vi "2023_day19.vi"() -> ()   [LabVIEW 2021]
uses:
  <vilib>/regexp/Match Regular Expression.xnode
panel:
  out "Task 1":i32
  out "Array":cluster{"Array":string[], "Array":i32[]}[](array[cluster])
  out "Rules":T1(array[cluster])
  out "line 2":string
  out "line":string
  in  "Switch":bool caption="Ex. Data  vs.  User Data"
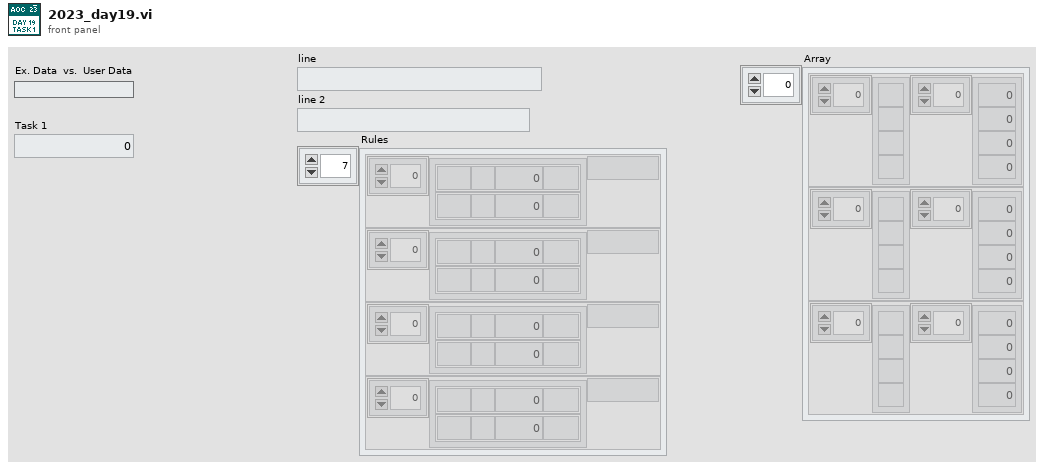
[diagram p1: front panel]
types:
  T1 = cluster{"Array":cluster{"String":string, "String":string, "Numeric":i32, "String":string}[], "String 2":string}[]
  T2 = cluster{cluster{string, string, i32, string}[], "delimiter (Tab)":string}
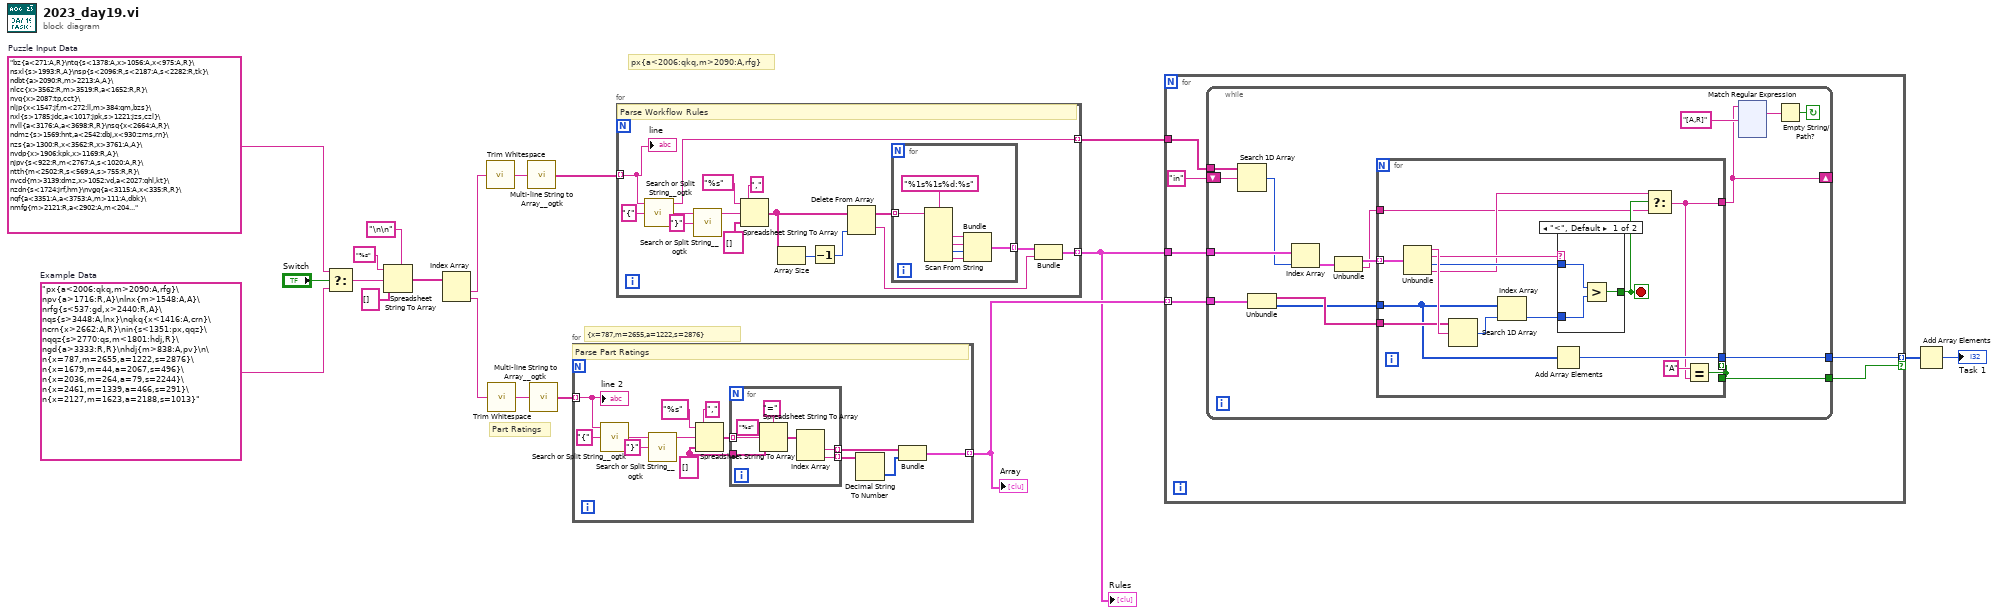
[diagram p0: block diagram]
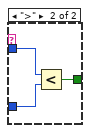
[diagram p2: hidden frame]
diagram:
  w17 = "bz{a<271:A,R}\ntq{s<1378:A,x>1056:A,x<975:A,R}\nsxl{s>1993:R,A}\nsp{s<2096:R,s<2187:A,s<2282:R,tk}\ndbt{a>2090:R,m>2213:A,A}\nlcc{x>3562:R,m>3519:R,a<1652:R,R}\nvq{x>2087:tp,cct}\nljp{x<1547:jf,m<272:ll,m>384:qm,bzs}\nxl{s>1785:jdc,a<1017:jpk,s>1221:jzs,czl}\nvll{a<3176:A,a<3698:R,R}\nsq{x<2664:A,R}\ndmz{s>1569:hnt,a<2542:dbj,x<930:zms,rn}\nzs{a>1300:R,x<3562:R,x>3761:A,A}\nvdp{x>1906:kpk,x>1169:R,A}\njpv{s<922:R,m<2767:A,s<1020:A,R}\ntth{m<2502:R,s<569:A,s>755:R,R}\nvcd{m>3139:dmz,x>1052:vd,a<2027:qhl,kt}\nzdn{s<1724:jrf,hm}\nvgq{a<3115:A,x<335:R,R}\nqf{a<3351:A,a<3753:A,m>111:A,dbk}\nmfg{m>2121:R,a<2902:A,m<2043:A,R}\nbxp{s>3412:A,m<2753:A,R}\nnxn{x<672:A,m>2353:A,R}\nhpr{a>1842:A,a>728:hcz,x>1243:A,A}\ncvl{a>669:mjv,m>2629:sc,rdf}\nkxx{a>766:R,a<292:R,A}\ndmg{s>2102:A,s>2014:A,A}\nrgv{a<3593:A,A}\nchn{a>2598:cbs,s>174:A,a<2260:tx,R}\nxz{m<1473:A,x>3212:R,x<2650:A,R}\ngzf{x>339:R,s>2706:R,A}\nzsr{a>3599:R,m>3283:R,s<1003:R,A}\nkc{m>1743:A,a>1102:R,x<2016:A,A}\nfns{s>2718:R,m<250:R,zz}\nrks{x>1085:A,a<3193:R,R}\ntsb{x>2609:R,R}\njpk{a<367:lmr,lkr}\nzt{x<728:A,x<1273:A,x<1612:A,R}\nsm{s<2016:R,m>3494:R,R}\nlqv{x>2509:rgv,mdj}\nqgc{s<2535:A,A}\nmn{x>711:R,R}\nqj{m<2321:A,a>1060:A,m<2640:A,A}\nlvl{x>2318:R,x>1150:R,R}\nfvj{x>629:xm,m>434:tg,R}\ndrm{x>3363:A,s<67:A,m<966:A,A}\nhc{a>2875:R,a<2355:R,A}\nrzh{x<2577:rt,a<1217:zjs,a<1672:A,xt}\nbcf{m<75:tm,s>2347:A,cjj}\nxsd{m<124:A,s>2385:A,bsn}\ndx{m<1166:R,A}\ncsf{s<815:sxq,a<2075:dck,ndb}\ndt{s<3903:R,a>3046:R,A}\nxbj{a<2484:bp,x>3289:rfz,s>239:vs,xs}\njmg{a<3045:pxt,lp}\nmpz{x<1593:R,x>3044:R,a<3808:A,A}\nlhp{x>1339:R,s<2653:A,x>649:R,A}\nll{s<3281:R,A}\ndcq{x>3360:R,m<3027:R,R}\nppg{m<541:R,m>559:R,x<2390:R,R}\nmbz{m<3495:R,s>2446:rks,A}\ncd{m<1335:A,m>1438:A,R}\nkrc{x<733:mfg,a>2761:qh,x>953:dch,zp}\nlvg{m>972:kz,x>495:hzn,a>3117:A,A}\nzhs{m>2206:rf,a<835:A,a>1165:R,R}\nfsh{x>2167:A,s>849:R,R}\nkbr{m<611:cpv,dp}\nrmx{a<1561:rs,s<1865:vq,m<710:tbz,fvq}\nhnh{s<2247:A,s>2348:R,m<339:R,R}\nhzq{m>626:A,a<2948:A,s<2726:A,R}\nrx{s<2136:A,s<2240:R,m>2747:A,R}\nqm{m>429:A,a>2633:dzg,a>2161:A,R}\nsbn{m<3741:R,m<3839:A,s<1462:A,R}\nlpk{s<3389:R,A}\npxt{a>2883:hzq,zh}\nfvq{s>2926:dvb,vmx}\nrz{s>425:md,s<168:pn,R}\nhxn{x>439:R,a<1407:A,A}\nqpg{m>3129:R,R}\npb{a>1824:vzm,x>3183:spc,qmb}\ndvj{a>925:R,s<234:A,R}\nksm{m>1071:A,m<396:A,s<327:A,R}\nqd{m>2276:R,s<225:R,x>3486:R,R}\njzs{m<2895:prh,s<1539:R,a>1512:ktn,zs}\ndp{x<1710:A,m<665:R,a>3405:R,R}\nfnf{s>2544:A,m<2240:R,A}\nfk{a>767:A,m<2071:R,R}\nndq{x<581:vr,a>2446:qjm,s>2111:jl,dhs}\nkkl{s>2054:R,m<3499:R,m<3761:R,cjk}\nxtv{a>1875:A,x>3752:R,m<2351:A,A}\nxpf{s<1203:nr,m<3594:vn,x<2455:A,sbn}\nhfx{a<1359:R,s<449:A,s>777:R,A}\nmrm{a>1753:tpl,x>1066:zzk,glm}\nnxx{s>2462:gxf,jz}\nqsf{a>2892:R,A}\nxt{s<1927:R,s<2188:A,a>1886:A,A}\nvbm{a<1287:A,xsj}\ncdh{a>2648:dq,vtq}\njc{m>2325:R,x<465:A,m>2139:A,R}\nzzk{a>1062:xg,m>3439:vf,lg}\nfvl{s>3488:R,a<3070:A,A}\nkdk{m>2643:gl,qd}\nbhd{x>1591:R,a<3099:R,R}\njdc{s<2074:dsl,m<2676:gc,A}\ngz{x>960:A,vgq}\nps{m>337:A,A}\nclf{s<1430:ct,nk}\nbsn{a<2452:R,s<2072:A,a<2687:A,A}\nfjr{s>918:zsr,m<2877:A,R}\nbx{m>3430:R,A}\nzg{m>1485:A,s>2852:A,m<1298:R,jrq}\nlp{x<1690:A,s>2595:R,x>2670:A,R}\nqmb{x<2671:lnl,s>696:R,A}\njk{s<1930:R,x<2990:R,R}\nlx{a<2583:dz,mbc}\npkq{s<368:R,s>527:R,a>3711:A,R}\nrzl{m>1462:A,s<2457:A,s<2597:R,R}\ntgr{a>2640:R,R}\npj{x>2209:xp,a>2278:A,mt}\nlmr{s>1359:R,x<3503:R,A}\nnq{x>1084:R,x>478:R,A}\nndb{a>3110:ss,x>3077:gmd,s<1734:fn,js}\nvpg{x<706:fdp,a>852:hfx,a<542:A,A}\ngxn{a<312:lsk,x>2287:dj,A}\ntcl{a>1665:A,zzr}\nsjk{x>3226:A,A}\nfkb{m>2795:jk,a<3439:jq,x>3038:R,bzr}\npl{m<1045:A,s<3912:A,x<2819:A,R}\nhhj{a>2420:R,s<2764:R,a<2288:R,A}\nsqb{s>1984:rx,R}\nqbd{m>2065:A,x<882:A,m<1999:R,A}\ngxv{m>595:R,a>3447:ppg,x<2625:R,fpx}\nbf{a<3541:R,drm}\nzjs{s<1967:R,s>2205:R,R}\ncct{s<720:hj,jqg}\nsqr{s<815:R,m>3766:R,s>962:A,A}\ndsl{a<888:A,m>3114:A,R}\nhg{a<3188:A,a<3272:A,R}\ngn{m<348:A,a>3297:R,A}\ncrq{m<369:cdk,x>1901:lh,gz}\nzzr{a>1577:R,s<2759:A,s>2978:A,R}\nsdq{s<2531:ft,nbf}\ncx{s<2002:A,A}\nzch{m<3110:A,a<580:R,A}\njm{a>3202:A,tth}\ntpl{m<3521:rp,s<417:chn,vgg}\nlsk{s<2835:A,a<146:A,A}\nkt{s>1824:gj,m<2677:jxf,gcz}\nvdb{s<2725:R,A}\nkrk{m>1118:A,x>3794:A,s<2745:A,A}\nhx{s>3398:R,s<3375:R,x<1299:A,A}\nmbc{x<3258:R,a>3221:R,x>3540:A,dcq}\nbcq{s<707:vvf,m<463:rv,A}\nvf{x<1370:R,s<575:A,sqr}\nmk{m>2037:tfj,x>1441:A,s<2719:A,A}\nktn{a>1844:R,x<3658:A,s>1639:A,R}\nhkh{s<3644:qnf,a>2509:R,a<2158:jg,sj}\nqkb{s>221:A,A}\nnbf{x>1635:A,R}\nktf{s<1930:jff,a>729:sv,s<2195:R,R}\ntbz{s>3054:hjn,m<295:ts,m>474:sf,rtk}\nrg{a>2237:A,s>2763:R,R}\ntn{s<2624:mq,vdp}\nzx{s<2597:R,R}\nhp{s>3853:dt,s<3725:nss,tgr}\nkkh{a>2790:R,m>189:A,R}\npmb{m<257:R,R}\ntx{s>78:R,a>2050:R,R}\nzhq{a>1619:A,x<2261:R,R}\nqh{m>2162:R,m>2032:A,R}\nsfh{s>3658:R,A}\nxs{x<2780:R,A}\nmv{a<2521:hd,gxv}\nzl{x>2215:cd,m>1293:hq,xv}\nqc{s<1635:A,A}\nvb{x>631:vkd,s>2815:xn,s>2755:A,gzf}\nlv{s>3494:A,A}\nlj{a<2530:A,m>36:R,A}\nkz{x>572:R,a<2969:R,A}\npnb{m<81:ljx,xsd}\nrv{s>1327:A,A}\nnkl{x>2711:R,x>2565:R,A}\ndkn{a<1500:pfp,x>1968:dtr,cpb}\nsz{m<2803:cfx,mbz}\nvm{s>3556:xtv,fg}\nvqr{a<2337:A,s>2233:R,R}\nss{s>1468:fkb,s<1048:fjr,x<3082:qfl,cjz}\nfp{a>2830:A,s<2169:R,R}\nrjr{m>1228:R,R}\nkl{a>644:A,R}\nzlb{x<1411:qf,a>3522:bcf,nxx}\nckr{m<2196:qbd,x>784:R,mxv}\nhb{m>2153:R,R}\nnml{x<1589:qv,sxk}\nqr{m<2677:A,s>2608:R,m<3452:A,A}\njh{s>1262:glg,m>2684:A,R}\nkh{m>2680:A,m>2361:R,A}\nvr{x<257:R,xhv}\nhjn{m>467:mv,s>3603:hp,ljp}\nfq{m>2822:tv,x<2595:nml,x<3261:tt,rfp}\nvtq{x>2240:xz,s>3083:A,dh}\ngb{s<2899:bz,tb}\nmrd{x>1271:lr,m<2641:rm,x<526:zqr,fs}\nmld{a>2486:A,x>3111:R,m<316:A,R}\nhcc{a<1236:A,a<1350:A,zlx}\nfs{s>603:R,A}\ncjz{a>3524:R,fjh}\npjk{a<2164:R,s<3627:R,x<2770:A,A}\nmxv{x<464:A,R}\nmjv{a>987:xhn,vtt}\npfc{s<3515:R,m<2266:A,s<3692:R,A}\ntz{m>914:kkg,a<2667:rng,x<1472:rq,gn}\nqhl{s<1607:jkc,a>1133:mds,nt}\nqg{s>1998:R,x<2415:A,R}\ndl{s<2694:ghj,x>2629:xpd,lqs}\nvgg{a>2972:R,zt}\nvqd{s>1429:A,x>354:A,A}\nqfh{s>3793:xpb,x<2138:hkh,a>2637:vg,hv}\nvmx{s>2326:dl,x>1382:dpd,m>1421:ndq,vrf}\nxsj{m>2720:R,a<1313:R,a>1330:A,R}\nnps{a<2079:R,m>1380:R,a>2173:kf,A}\nkxp{m<1582:A,A}\njln{m<1242:A,a<2086:R,a>2252:A,A}\ntfj{a>392:R,x>1464:A,x<774:R,R}\nghj{m<1275:vnz,m<1584:rzl,m<1710:hc,lvl}\njmb{s>2167:R,s>2124:R,R}\njg{x<1043:R,R}\ngc{m>2288:R,x>3485:R,A}\nlch{m>981:A,x<307:A,A}\ndch{m<2204:R,a>2068:R,R}\nfj{a<855:zg,gvv}\nhv{m>1308:pjk,a>1953:R,m>961:R,sfh}\ntv{a<1389:ctq,pj}\nqt{m>3033:ktf,m>2364:sqb,rzh}\ndhs{m<1658:A,s>1977:sft,x>884:R,xdl}\nbld{x<2869:A,R}\nlh{m<436:dbl,a<2712:lq,m>457:A,A}\nhvh{s<242:R,m>1756:hqt,x<1329:A,dzs}\nzb{x<902:R,s>341:A,s<172:A,R}\nmd{a>3376:R,R}\nzlx{s<733:A,R}\nxcl{a>870:A,m>3355:A,a<455:R,R}\nvmn{s<2480:A,R}\nhqt{a<526:A,m>1813:A,R}\ntnp{s<1812:R,bgn}\nljx{x<2542:lhp,lj}\npg{x<1652:R,R}\nvd{x<1464:hpr,x<1655:tnp,sxn}\nzh{m>578:A,a<2830:A,R}\ndzs{x>1651:A,A}\nsj{s<3698:R,m<1133:A,A}\nks{a>1809:A,R}\nxpb{x<1450:R,m>1232:zq,pl}\nffg{x>2163:lt,s>3351:hx,x>786:qnr,lch}\ndnn{m<2585:R,A}\ngmd{x<3605:zdn,gct}\njq{x<2628:A,A}\ncpv{s<2035:R,R}\ngct{x<3764:A,x>3852:R,a>2497:hl,A}\nvlc{x>2214:A,s<3472:R,s>3806:A,A}\nbvl{m<2738:R,R}\nvxf{m<3019:A,x<3541:A,A}\ntg{a<3439:R,s<2677:R,R}\nfsf{a>2519:A,R}\npv{a<420:A,m>1733:A,R}\nfff{a>2742:A,x>3397:A,A}\nlb{s<2419:A,s<2498:R,a<1250:A,R}\ngfp{x>3062:A,A}\ncjj{a>3731:R,A}\ndqf{s<2041:R,a<2123:A,vpk}\npc{x<2498:R,s>2942:A,R}\npsb{m<380:A,m<422:rjp,R}\nxhn{m<2996:qj,a>1071:cn,a<1022:R,hgp}\npt{a<2754:nkl,A}\nzjz{a<734:A,R}\npm{x<1100:A,m>2655:R,a>3140:R,A}\nrdf{m>2278:gxn,x>2317:cvv,mk}\ndts{x>1531:pg,a<3446:vj,m>1041:kq,pkq}\ndck{x>3214:xl,s>1666:qt,nsj}\nlc{x>361:A,A}\nkkg{m>1303:A,a<2452:A,x<1273:R,R}\nvg{x>3184:A,m<1418:R,x>2660:bld,A}\njt{x>2477:R,a>2635:zx,fsf}\nhm{a>2487:A,a<2274:A,m<2628:R,R}\ngdf{a>1833:A,m>2601:R,x>3693:A,A}\nbn{s>2146:A,R}\nmds{a<1669:kh,ks}\nkjs{m<1076:bg,x<2959:sq,a>2348:jzk,nps}\ntpd{m>3019:R,m<2929:zjz,dhm}\nvj{a<3135:R,A}\nin{m<1904:rmx,dv}\nbg{x<2803:zk,A}\nkq{s>335:R,x<1444:R,s<144:R,R}\ndh{m<1504:A,x<1117:R,R}\nglg{s>1491:A,a>2699:R,x<2115:R,R}\ngq{m>582:A,s>2494:R,R}\nczl{m>3218:lcc,a>1482:gdf,s>1070:R,jpv}\nfb{x<798:A,m<1278:A,x<1320:A,R}\nbgn{m<2676:A,x>1552:A,a<2102:A,R}\njkc{s>1316:lvr,A}\njff{s<1814:A,A}\npfp{a>1356:lk,s<2593:lb,vbm}\nhzn{s>291:A,m<350:R,s>107:A,R}\nnss{x>1361:R,m<275:R,A}\nmt{a>1794:A,a<1619:A,R}\ncbs{x>749:R,x>452:A,R}\nzp{a>2382:R,m>2160:A,A}\ncdj{m<1426:A,m<1470:R,R}\ngkc{a>3431:A,m<2719:R,R}\nrng{a<2253:A,s<1364:A,A}\ncm{x<701:A,s<2077:R,R}\nsl{s>218:A,a<1428:R,R}\nlr{s<676:dnn,m<2639:R,tkc}\nqrj{a>3647:A,R}\nqfl{x<2572:pf,x<2780:R,a<3582:A,lzt}\nkd{a>2021:R,x<3445:R,A}\nhth{a<436:bj,a<537:A,a>618:rd,zch}\nvtp{m>2029:fk,s<186:A,fv}\nlk{x>1877:R,x<1197:hxn,s>2758:mg,qr}\nfjh{s<1233:A,s>1369:A,A}\nbl{x>3051:kdk,m>2606:cs,x>2593:qkb,dqk}\njxc{s<754:A,s<919:R,x>326:R,A}\nsh{m<1271:ffg,x<2154:lpk,ml}\nrvk{a>1716:jb,m>2310:mrd,x<929:bsr,mtv}\njz{s<2076:A,R}\ngxf{m>119:R,R}\ntm{s>2460:R,s<2108:A,R}\nhs{a<1050:A,s>1331:A,A}\nklm{m>334:A,a<3340:hg,mn}\nvrf{x>831:qn,jss}\ntk{x<714:R,m>536:A,A}\ngcz{x>689:fgq,a>2814:R,a>2515:R,R}\nvrc{a>617:hcc,bcq}\nfv{x<323:A,a>731:R,m<1985:R,R}\nqv{s<3495:nxn,ntn}\nzqr{s>620:R,a>1126:bvl,a>521:klf,pht}\nhcz{m>2716:R,a<1342:A,s<1707:A,R}\nxn{s<2868:R,A}\nph{a<420:A,x<2533:R,a<671:R,A}\nbp{a>1918:A,x<3035:rjr,m<1071:xzr,R}\nzdf{a>958:A,pv}\nhgp{a>1049:R,R}\nmq{m>638:A,s<2293:A,a>616:pmb,ql}\ncn{s<2663:A,R}\ndhm{s>353:A,R}\njzk{s<568:R,x>3650:A,s>707:R,R}\ncjk{x>2540:R,s>1858:A,m>3890:A,A}\ncrx{m>562:gq,x<1668:mf,x<2473:R,qgc}\nbjh{s>952:A,R}\nfxm{x<480:R,a<2492:A,x>663:dtc,cdt}\nvfp{x<2978:R,s<2782:R,bx}\nklf{s<297:R,A}\nrm{a<641:vv,R}\nflb{s<2029:R,A}\nvnz{a>2624:A,R}\nfth{m<3233:A,x>2427:A,a<1264:R,R}\nqzc{s<2056:fd,x<2546:jmb,fp}\nxzr{a<1702:A,x<3487:R,R}\nspc{x<3466:A,R}\nrvs{m<2531:R,s<732:R,a>1885:R,A}\nbj{x<2674:R,x<3312:A,R}\nctq{x>2179:ktg,xcl}\nljf{a>2607:R,A}\nsxk{a<2523:vlc,a<3269:nlv,pfc}\nvkd{m<3011:R,A}\nfpx{x<3400:R,m<513:A,m<550:R,A}\njvz{x<2305:R,R}\ntp{s>785:clf,a>3143:fc,s>403:kjs,xbj}\nbzr{x>2399:A,A}\nct{s<1142:R,m>1072:cxn,m<576:R,R}\ndpz{x<2890:R,m<1145:R,m>1208:A,R}\ntdk{s<953:R,s<1004:A,A}\nvvf{a>308:R,R}\nmdc{s<545:A,R}\nzms{s<1338:vt,vqd}\nsxq{s<539:bl,pb}\nnpq{a>1733:A,s<2028:R,A}\nst{s>1119:kkn,a<1471:fth,a>1798:A,A}\nqgx{s<2114:qg,x<2550:dx,kd}\ntkc{s<834:A,s>935:R,s<888:A,R}\nvn{a>368:A,x>2719:R,a<186:A,R}\nhdj{m>1379:R,a<3199:A,R}\nfdk{s>760:R,s<721:R,R}\njss{x<523:A,m>949:ljf,cf}\nhfj{m<2440:R,A}\nxmq{s>721:A,A}\nglr{s<409:R,a>2481:vx,a<2006:rvs,R}\npn{s>103:A,x<1962:R,x<2041:R,R}\nrbn{m>1175:A,x<1104:R,A}\nkxh{s>260:A,R}\ngj{x<583:R,R}\nxhd{m>1531:A,x<2769:A,A}\nln{x>1465:R,m>3662:R,A}\nkj{a>2600:R,a>2074:R,a<1875:A,R}\nrds{s>3324:R,m>318:R,A}\ndg{s<1209:R,x<1771:A,a<1172:R,R}\ndj{m>2401:A,x<3015:A,R}\nxcs{m>1181:A,qrj}\nnr{x>2543:R,R}\njrf{s<1411:A,x>3427:A,a>2442:A,A}\nmm{x<803:R,x>1048:A,R}\nts{m>185:nz,a<3026:pnb,zlb}\nnz{a>2521:jzb,s>2272:fns,dqf}\njqg{x>791:tz,fxm}\nrfz{m<1244:R,m>1510:A,m<1357:A,cdj}\nmg{a<1429:A,A}\nlld{a<2189:R,x<1847:R,x>3023:A,A}\nfql{a>1962:A,A}\nfc{s>306:xcs,s<188:bf,a>3705:kxh,knl}\nqhm{a>3166:R,x<2392:R,s>2102:A,A}\nbzs{s>3380:vll,s<3197:tsb,s>3273:rds,mld}\nxxf{x>1829:lx,s>2658:ljc,sz}\nmf{a<3800:R,A}\nnk{a>2593:qc,hxg}\nxsx{a<1715:A,a<1733:A,R}\nsf{s<2353:fx,a<2799:cgr,a>3459:jj,jmg}\nlg{a<481:R,m<3125:mdc,A}\nlqs{s>2841:A,x>1238:A,a>2711:R,rg}\ncdt{s>1120:R,s<974:R,m<793:R,A}\ncgr{a>2377:jt,fql}\nvv{m>2422:R,A}\npht{x>323:R,m<2739:R,s<391:A,A}\nfd{s<1901:A,x>2345:R,R}\nqnf{x>1052:A,A}\nslf{x<2902:A,x<3031:hb,a>1612:xb,R}\nrp{a<2688:qpg,s<561:zb,s>820:bjh,xmq}\nxp{x<3009:A,s>3497:R,R}\nsc{s<2609:vmn,x>1372:hth,gb}\nxb{x<3182:R,m>2184:A,m<2037:R,R}\nntn{m>2269:A,A}\nvpk{a<2369:R,m<252:A,x<2607:A,R}\nvx{m<2559:R,R}\nrjp{s<2679:A,a<2465:R,s<2825:A,A}\nms{m<1237:dg,a>1188:R,s>1186:hs,fsh}\nvt{a>3078:A,m>3607:A,s<1211:R,R}\ndf{m<2520:A,A}\nsft{a>1928:R,A}\nhq{x>1359:R,m>1393:R,R}\ndd{s<3456:jlj,A}\nfph{s>1556:fj,s<564:ls,m<1556:hxz,zmf}\nrs{m<1078:srt,fph}\nktg{s>3470:R,R}\nzk{m<406:R,a>2584:A,R}\nqjm{m>1597:A,s>2130:vfr,m>1500:cx,sxl}\nzz{s>2430:A,A}\njl{m<1587:A,a<2096:R,a<2280:R,vqr}\nvmt{m<3197:R,x<2588:R,x<2868:sm,R}\nbk{x<2404:A,x>3166:R,A}\nmdj{x<1270:A,A}\ngk{x<2248:A,x<2842:A,A}\nnt{m<2598:jc,x<407:A,s>1913:cm,R}\nzkj{m<2762:qsf,s<609:R,mm}\nfgq{x<850:A,a<3052:A,A}\nvfr{a>3009:R,A}\nxm{a>3477:A,m>406:R,x<960:A,R}\nkkn{x<2769:A,a<1377:R,x<3030:A,R}\ncf{x<659:R,x>729:A,A}\nzmf{x>1721:zdf,rfj}\nxpd{x<3509:R,s>2838:A,krk}\ncq{m<808:A,s>2073:A,R}\nxg{s>399:A,x>1421:A,sl}\nlt{m<933:A,s<3372:R,s>3403:R,R}\nrf{m<2272:A,a>1003:R,s>202:A,A}\nbqd{a<3165:kj,rql}\nlms{a>1748:A,s>2636:xsx,m<2315:R,df}\nlkr{x<3666:R,R}\ndvb{s>3461:qfh,s<3266:cdh,sh}\nlvr{x<596:R,a>821:R,R}\nxhv{s>2049:A,A}\nxdl{s>1934:A,a<2067:R,s>1892:A,A}\ndbl{s>2134:R,s<1998:R,R}\nsrt{s>1912:tn,vrc}\nzq{x<2350:R,m<1616:R,A}\nzpc{m<3078:nq,R}\nql{x<2222:R,a>217:A,m>243:R,A}\ncs{m<3468:A,s<268:R,s>406:shg,nrp}\nkp{a<604:R,A}\njzb{a<3429:A,A}\nls{x>2029:xhd,m>1549:hvh,tf}\nqnr{m>1000:A,R}\ndq{s<3056:hdj,s>3189:gk,m<1420:A,A}\ntb{s>2981:R,m<3206:A,A}\nglm{m>3351:vpg,tpd}\nqsm{m<1972:A,m<2023:A,s<2691:A,R}\nft{x<2027:A,x>2763:A,R}\nrn{x>1317:bhd,x<1173:tq,A}\ndqk{x>2356:dbt,x>2136:zhq,a>1610:R,A}\nnv{x>1361:bqd,a<2999:psb,m>357:fvj,klm}\njxf{m>2189:hfj,A}\njs{a<2660:vmt,m>3052:kkl,qzc}\nkpk{x<3286:A,x>3662:R,R}\nqn{s>2152:R,s>2016:rbn,A}\nkf{s>585:A,m>1213:R,A}\nknl{x>2896:R,jr}\nprh{a<1460:A,A}\njrq{a<426:R,a>638:R,R}\ngl{x<3393:A,s<287:A,A}\nfdp{x>267:A,s>393:R,A}\nbsr{s>376:ncs,m<2142:vtp,zhs}\nshg{s<469:A,x<2595:A,R}\nctz{m<2081:fdk,kxx}\nnl{s<2520:A,m>2555:A,x<3105:R,R}\nsxn{a>2415:gkc,R}\ndbj{a>1076:R,a<489:R,A}\nljc{s<2911:vb,zpc}\nfmg{x<1058:bn,a<2339:R,x>1297:A,A}\nrfp{x<3517:dd,vm}\npx{a<465:A,a>714:A,R}\ndzg{s>3282:A,s<3184:R,s>3219:R,A}\nlq{x>3134:A,R}\nxv{s<919:A,a>320:R,s<1148:A,R}\ndtq{x<2179:A,x>2391:ph,A}\nlzt{s>1227:A,R}\nrq{m<349:A,A}\nrtk{s<2469:crq,nv}\ndv{s>2329:pqs,x>1932:csf,zn}\nvs{x<2598:ksm,qcr}\ndpd{a<2738:qgx,m>1283:bbc,ffl}\nrt{s>1987:R,m>2159:R,m>2063:A,R}\ndtc{x<745:A,a>3398:A,m<1224:A,R}\nrfj{s<990:kl,A}\nrd{x<2353:R,a<648:R,x>3265:A,R}\nxdm{x<1258:R,x>1548:A,R}\nrmg{a>1998:R,s>2112:A,flb}\nbv{s>774:R,x<3030:A,R}\nfn{x>2408:pt,jh}\ntt{m>2448:kbj,slf}\ndz{a<2220:A,hhj}\nml{x>2990:fff,a<2565:R,kxp}\nhd{m<570:lld,a<1904:lv,x<1590:A,bk}\nhxg{x<3092:A,m>1196:R,s<1660:R,R}\ncxn{x>3190:A,m<1403:A,s>1314:A,R}\njb{x>1245:jm,m<2402:krc,m>2698:zkj,glr}\npf{s<1266:A,m<2902:R,x>2251:R,R}\nhj{x<1378:lvg,a<2521:jln,x>1817:rz,dts}\ncpb{m>3169:dnk,m<2567:ckr,tcl}\ndbk{m<56:R,x>700:A,a>3875:A,R}\npqs{s>3117:fq,a>1848:xxf,a>1154:dkn,cvl}\nnlv{a<2823:A,a>3076:R,a>2987:R,R}\nvtt{a>783:vdb,m<3188:R,s>2709:pc,A}\nfx{a>2764:kbr,x>1635:rmg,m<589:sp,fmg}\nnrp{a<1932:A,x>2604:A,a>3260:A,A}\nsv{x>2615:R,s<2155:R,A}\ncvv{m<2065:qsm,s<2757:R,R}\ngvv{m<1550:R,kc}\nhl{m>3176:A,x<3803:A,R}\nrql{x>2295:A,s>2830:A,A}\njf{s<3352:kkh,m>311:R,m<107:fvl,R}\nhxz{a>804:ms,zl}\nncs{x>559:A,m>2043:lc,a<640:A,jxc}\njlj{s>3247:A,A}\nffl{m<928:cq,a>3573:dpz,m>1062:A,qhm}\ncfx{m<2449:fnf,pm}\nbbc{m>1669:A,m<1442:jvz,x<2353:dmg,gfp}\nfg{x<3812:R,m>2492:A,A}\njr{a>3444:R,a<3293:R,A}\ndnk{m>3704:xdm,A}\ndtr{m>2899:vfp,a>1679:lms,knr}\nnsj{a>1009:st,m>2813:xpf,x<2635:dtq,px}\nlnl{x>2417:A,A}\nhnt{x<1231:npq,ln}\ntf{a>536:dvj,fb}\nqcr{x>3055:R,A}\nkbj{m<2677:A,bxp}\njj{s>2662:mpz,m>609:sdq,a>3669:crx,lqv}\nmtv{s<699:kp,s<859:ctz,tdk}\nvzm{s>714:bv,s<612:A,x<3205:R,vxf}\nzn{s>1050:vcd,m<2850:rvk,mrm}\ncdk{x<2570:hnh,a>2692:R,s<2088:A,ps}\nknr{s>2839:sjk,s>2584:A,s<2459:A,nl}\n\n{x=1464,m=163,a=691,s=469}\n{x=61,m=72,a=436,s=2532}\n{x=358,m=100,a=2631,s=347}\n{x=266,m=439,a=1250,s=358}\n{x=81,m=2110,a=30,s=86}\n{x=1224,m=758,a=1133,s=881}\n{x=1391,m=3763,a=16,s=2076}\n{x=1149,m=1148,a=126,s=3270}\n{x=214,m=590,a=492,s=818}\n{x=1305,m=687,a=737,s=90}\n{x=20,m=75,a=868,s=847}\n{x=1588,m=99,a=2314,s=998}\n{x=360,m=1002,a=33,s=164}\n{x=68,m=1589,a=992,s=691}\n{x=740,m=2150,a=691,s=668}\n{x=2165,m=707,a=1189,s=161}\n{x=158,m=53,a=416,s=1124}\n{x=601,m=217,a=962,s=623}\n{x=2,m=1314,a=1150,s=357}\n{x=2931,m=1911,a=54,s=1046}\n{x=1037,m=1,a=78,s=974}\n{x=2460,m=689,a=1003,s=1253}\n{x=1793,m=1250,a=331,s=306}\n{x=243,m=247,a=156,s=146}\n{x=1380,m=1600,a=387,s=1362}\n{x=35,m=1900,a=38,s=411}\n{x=349,m=118,a=2452,s=143}\n{x=1314,m=2751,a=1835,s=1569}\n{x=51,m=950,a=1436,s=376}\n{x=347,m=2004,a=11,s=537}\n{x=490,m=576,a=484,s=3066}\n{x=1,m=891,a=3506,s=446}\n{x=1994,m=519,a=644,s=1335}\n{x=2230,m=1165,a=391,s=630}\n{x=1606,m=853,a=1668,s=371}\n{x=904,m=602,a=632,s=1969}\n{x=583,m=794,a=2018,s=851}\n{x=938,m=373,a=1253,s=104}\n{x=704,m=514,a=617,s=525}\n{x=366,m=1662,a=33,s=314}\n{x=753,m=1002,a=285,s=170}\n{x=959,m=2924,a=65,s=1249}\n{x=222,m=701,a=8,s=610}\n{x=887,m=350,a=209,s=3369}\n{x=467,m=137,a=80,s=267}\n{x=671,m=1325,a=928,s=2499}\n{x=69,m=1915,a=539,s=277}\n{x=119,m=2442,a=482,s=495}\n{x=339,m=2398,a=1553,s=1128}\n{x=1364,m=1330,a=1025,s=1678}\n{x=527,m=325,a=341,s=602}\n{x=309,m=1764,a=2066,s=1672}\n{x=772,m=102,a=110,s=723}\n{x=407,m=1522,a=2722,s=26}\n{x=286,m=426,a=863,s=1849}\n{x=483,m=1557,a=1569,s=74}\n{x=487,m=3225,a=2582,s=2012}\n{x=46,m=39,a=650,s=2371}\n{x=98,m=1618,a=1354,s=1140}\n{x=143,m=1488,a=2612,s=3212}\n{x=1894,m=6,a=301,s=2723}\n{x=880,m=50,a=1989,s=1331}\n{x=899,m=308,a=3250,s=1097}\n{x=6,m=235,a=868,s=246}\n{x=128,m=1556,a=1238,s=746}\n{x=561,m=1864,a=743,s=17}\n{x=1170,m=525,a=473,s=2178}\n{x=1927,m=581,a=164,s=1762}\n{x=2467,m=1688,a=258,s=223}\n{x=91,m=80,a=2047,s=1}\n{x=592,m=261,a=374,s=2523}\n{x=1624,m=507,a=3574,s=2063}\n{x=1299,m=696,a=861,s=2958}\n{x=521,m=188,a=1693,s=1079}\n{x=184,m=570,a=1080,s=3064}\n{x=895,m=188,a=714,s=93}\n{x=488,m=123,a=4,s=1884}\n{x=174,m=231,a=499,s=2306}\n{x=1309,m=1190,a=629,s=1364}\n{x=3901,m=1901,a=3133,s=806}\n{x=104,m=3125,a=420,s=80}\n{x=1108,m=13,a=118,s=1537}\n{x=79,m=228,a=1099,s=1009}\n{x=151,m=1805,a=439,s=158}\n{x=1140,m=26,a=358,s=254}\n{x=33,m=859,a=1798,s=2119}\n{x=1351,m=875,a=154,s=1526}\n{x=193,m=1105,a=181,s=273}\n{x=1669,m=697,a=3436,s=2059}\n{x=2207,m=1038,a=3441,s=17}\n{x=1619,m=451,a=126,s=613}\n{x=179,m=925,a=61,s=1001}\n{x=377,m=489,a=516,s=2503}\n{x=1234,m=254,a=1687,s=1737}\n{x=157,m=243,a=807,s=2647}\n{x=2085,m=2178,a=1890,s=2279}\n{x=2543,m=41,a=1601,s=958}\n{x=491,m=651,a=1024,s=147}\n{x=1728,m=2320,a=1243,s=2661}\n{x=3255,m=52,a=300,s=12}\n{x=454,m=17,a=328,s=3}\n{x=25,m=2552,a=1744,s=2031}\n{x=914,m=1956,a=2626,s=537}\n{x=70,m=1644,a=1296,s=3639}\n{x=183,m=105,a=1468,s=729}\n{x=1054,m=817,a=54,s=797}\n{x=303,m=26,a=54,s=2919}\n{x=426,m=425,a=2235,s=290}\n{x=3366,m=1016,a=249,s=1868}\n{x=553,m=1259,a=1205,s=1739}\n{x=381,m=92,a=1879,s=1959}\n{x=340,m=2787,a=697,s=1705}\n{x=967,m=174,a=119,s=125}\n{x=2039,m=128,a=1808,s=187}\n{x=610,m=3225,a=159,s=133}\n{x=655,m=584,a=1571,s=1545}\n{x=453,m=2305,a=2208,s=1144}\n{x=264,m=2748,a=54,s=3012}\n{x=1780,m=1205,a=85,s=731}\n{x=994,m=538,a=2258,s=122}\n{x=721,m=293,a=116,s=1491}\n{x=92,m=871,a=938,s=1245}\n{x=824,m=66,a=217,s=1124}\n{x=1386,m=2328,a=22,s=1487}\n{x=134,m=208,a=3476,s=103}\n{x=2079,m=956,a=696,s=1512}\n{x=330,m=685,a=640,s=1277}\n{x=828,m=178,a=149,s=861}\n{x=1803,m=1792,a=3530,s=1056}\n{x=490,m=146,a=606,s=1823}\n{x=1095,m=12,a=1532,s=2254}\n{x=956,m=549,a=1656,s=2066}\n{x=589,m=129,a=377,s=1081}\n{x=703,m=423,a=1326,s=692}\n{x=1962,m=554,a=3730,s=403}\n{x=805,m=13,a=2957,s=435}\n{x=1014,m=1169,a=877,s=1628}\n{x=231,m=1783,a=3029,s=450}\n{x=2631,m=1113,a=2281,s=598}\n{x=1253,m=689,a=1380,s=269}\n{x=1218,m=257,a=693,s=1838}\n{x=2592,m=157,a=2692,s=2610}\n{x=182,m=1834,a=2526,s=2412}\n{x=7,m=2186,a=1092,s=2759}\n{x=378,m=2142,a=223,s=2671}\n{x=4,m=1224,a=1,s=1266}\n{x=362,m=665,a=1354,s=1927}\n{x=938,m=1440,a=779,s=451}\n{x=653,m=861,a=782,s=69}\n{x=1917,m=1353,a=2782,s=493}\n{x=768,m=226,a=774,s=2560}\n{x=2358,m=129,a=916,s=2}\n{x=1437,m=57,a=2611,s=535}\n{x=1620,m=713,a=399,s=975}\n{x=925,m=1213,a=196,s=40}\n{x=2587,m=1109,a=403,s=614}\n{x=2329,m=1563,a=2339,s=221}\n{x=1135,m=1141,a=2005,s=660}\n{x=336,m=831,a=244,s=561}\n{x=1860,m=527,a=1251,s=4}\n{x=108,m=3112,a=467,s=1376}\n{x=1024,m=1249,a=291,s=289}\n{x=1016,m=2544,a=380,s=681}\n{x=1029,m=2456,a=140,s=1858}\n{x=1896,m=86,a=814,s=2106}\n{x=948,m=2199,a=1919,s=1537}\n{x=1073,m=304,a=770,s=824}\n{x=1495,m=735,a=355,s=208}\n{x=775,m=118,a=105,s=132}\n{x=94,m=686,a=2362,s=1493}\n{x=663,m=202,a=89,s=1471}\n{x=415,m=285,a=639,s=594}\n{x=357,m=1340,a=558,s=686}\n{x=375,m=1342,a=875,s=323}\n{x=951,m=600,a=172,s=1109}\n{x=607,m=161,a=1132,s=327}\n{x=1158,m=117,a=360,s=1463}\n{x=813,m=2117,a=497,s=1136}\n{x=37,m=1790,a=644,s=174}\n{x=1744,m=133,a=1954,s=24}\n{x=1701,m=466,a=939,s=132}\n{x=2230,m=1484,a=287,s=46}\n{x=883,m=3196,a=1629,s=523}\n{x=40,m=2274,a=2969,s=1136}\n{x=2391,m=25,a=1371,s=598}\n{x=476,m=1117,a=678,s=1095}\n{x=515,m=1488,a=265,s=1929}\n{x=2765,m=325,a=834,s=826}\n{x=717,m=5,a=1380,s=4}\n{x=45,m=5,a=526,s=558}\n{x=756,m=3112,a=1,s=721}\n{x=388,m=760,a=635,s=2132}\n{x=2335,m=987,a=4,s=1253}\n{x=201,m=1422,a=2646,s=166}\n{x=585,m=684,a=146,s=522}\n{x=2358,m=998,a=1386,s=1620}\n{x=844,m=379,a=2917,s=903}\n{x=2701,m=3418,a=1938,s=1538}\n{x=1603,m=357,a=2232,s=2683}\n{x=3046,m=3073,a=194,s=169}"  # Puzzle Input Data
  w18 = "px{a<2006:qkq,m>2090:A,rfg}\npv{a>1716:R,A}\nlnx{m>1548:A,A}\nrfg{s<537:gd,x>2440:R,A}\nqs{s>3448:A,lnx}\nqkq{x<1416:A,crn}\ncrn{x>2662:A,R}\nin{s<1351:px,qqz}\nqqz{s>2770:qs,m<1801:hdj,R}\ngd{a>3333:R,R}\nhdj{m>838:A,pv}\n\n{x=787,m=2655,a=1222,s=2876}\n{x=1679,m=44,a=2067,s=496}\n{x=2036,m=264,a=79,s=2244}\n{x=2461,m=1339,a=466,s=291}\n{x=2127,m=1623,a=2188,s=1013}"  # Example Data
  # "{x=787,m=2655,a=1222,s=2876}"
  # "px{a<2006:qkq,m>2090:A,rfg}"
  # "Part Ratings"
  n1 = Select(t=w17, s="Switch", f=w18) -> (s? t:f=w16:string)
  n2 = Spreadsheet String To Array(delimiter (Tab)="\n\n", format string="%s", spreadsheet string=w16, array type (2D Dbl)=string[] []) -> (array=w13:string[])
  n3 = Index Array(array=w13) -> (element #1=w12:string, element #2=w11:string)  [unwired: 2 in]
  n4 = call <vilib>:"Trim Whitespace.vi"("string"=w12) -> ("trimmed string"=w9:string)  [unwired: 1 in]
  n5 = call <vilib>:"Trim Whitespace.vi"("string"=w11) -> ("trimmed string"=w8:string)  [unwired: 1 in]
  n6 = call <userlib>:"Multi-line String to Array__ogtk.vi"("string"=w9) -> ("lines"=w7:string[])
  n7 = call <userlib>:"Multi-line String to Array__ogtk.vi"("string"=w8) -> ("lines"=w6:string[])
  n8 = for {
    tunnel: w6 -> [w26] mode=indexing
    tunnel: [w20] -> w5 mode=indexing
    w24 = string[] [] ("array type (2D Dbl)")
    # "Parse Part Ratings"
    n9 = call <userlib>:"Search or Split String__ogtk.vi"("search string/char (-)"="{", "string"=w26) -> ("substring after match"=w31:string)  [unwired: 1 in, 2 out]
    n10 = call <userlib>:"Search or Split String__ogtk.vi"("search string/char (-)"="}", "string"=w31) -> ("substring before match"=w32:string)  [unwired: 1 in, 2 out]
    n11 = Spreadsheet String To Array(delimiter (Tab)=",", format string="%s", spreadsheet string=w32, array type (2D Dbl)=w24) -> (array=w25:string[])
    n12 = for {
      tunnel: w25 -> [w39] mode=indexing
      tunnel: w24 -> [w37]
      tunnel: [w34] -> w21 mode=indexing
      tunnel: [w33] -> w23 mode=indexing
      n13 = Spreadsheet String To Array(delimiter (Tab)="=" ("search string"), format string="%s", spreadsheet string=w39, array type (2D Dbl)=w37) -> (array=w35:string[])
      n14 = Index Array(array=w35) -> (element #1=w34:string, element #2=w33:string)  [unwired: 2 in]
    }
    n15 = Decimal String To Number(string=w23) -> (number=w22:i32[])  [unwired: 2 in, 1 out]
    n16 = Bundle(w21, w22) -> (w20:cluster{string[], i32[]})  [unwired: 1 in]
    "line 2" <- w26
  }
  "Array" <- w5
  n17 = for {
    tunnel: w7 -> [w47] mode=indexing
    tunnel: [w51] -> w3 mode=indexing
    tunnel: [w40] -> w4 mode=indexing
    # "Parse Workflow Rules"
    n18 = call <userlib>:"Search or Split String__ogtk.vi"("search string/char (-)"="{", "string"=w47) -> ("substring after match"=w48:string, "substring before match"=w40:string)  [unwired: 1 in, 1 out]
    n19 = call <userlib>:"Search or Split String__ogtk.vi"("search string/char (-)"="}", "string"=w48) -> ("substring before match"=w46:string)  [unwired: 1 in, 2 out]
    n20 = Spreadsheet String To Array(delimiter (Tab)=",", format string="%s", spreadsheet string=w46, array type (2D Dbl)=string[] []) -> (array=w44:string[])
    n21 = Array Size(array=w44) -> (size(s)=w43:i32)
    n22 = Decrement(x=w43) -> (x-1=w42:i32)
    n23 = Delete From Array(array=w44, index=w42) -> (deleted portion=w41:string, array with subset deleted=w45:string[])  [unwired: 1 in]
    n24 = for {
      tunnel: w45 -> [w62] mode=indexing
      tunnel: [w56] -> w52 mode=indexing
      n25 = Scan From String(format string="%1s%1s%d:%s", input string=w62) -> (output 1=w60:string, output 2=w59:string, output 3=w58:i32, output 4=w57:string)  [unwired: 6 in, 3 out]
      n26 = Bundle(w60, w59, w58, w57) -> (w56:cluster{string, string, i32, string})  [unwired: 1 in]
    }
    n27 = Bundle(w52, "delimiter (Tab)"=w41) -> (w51:T2)  [unwired: 1 in]
    "line" <- w47
  }
  "Rules" <- w3
  n28 = for {
    tunnel: w5 -> [w66] mode=indexing
    tunnel: w4 -> [w67]
    tunnel: w3 -> [w68]
    tunnel: [w64] -> w2 mode=indexing if=w63
    n29 = while {
      tunnel: w68 -> [w83]
      tunnel: w67 -> [w81]
      tunnel: w66 -> [w79]
      shift-right: [w73] -> _
      shift-left: "in" ("element") -> [w82]
      tunnel: [w70] -> w64
      tunnel: [w69] -> w63
      stop <- w72 continue-if-true
      n30 = Search 1D Array(1D array=w81, element=w82) -> (index of element=w80:i32)  [unwired: 1 in]
      n31 = Unbundle(w79) -> (w77:string[], w76:i32[])
      n32 = Index Array(array=w83, index=w80) -> (element=w84:T2)
      n33 = Unbundle(w84) -> (w78:cluster{string, string, i32, string}[], "delimiter (Tab)"=w71:string)
      n34 = for {
        tunnel: w78 -> [w216] mode=indexing
        tunnel: w77 -> [w214]
        tunnel: w76 -> [w209]
        tunnel: [w203] -> w73
        tunnel: [w208] -> w70 if=w202
        tunnel: w71 -> [w204]
        tunnel: [w202] -> _ mode=indexing
        tunnel: [w202] -> w69
        stop <- w205 stop-if-true
        n35 = Unbundle(w216) -> (w215:string, w212:string, w210:i32, w206:string)
        n36 = Search 1D Array(1D array=w214, element=w215) -> (index of element=w213:i32)  [unwired: 1 in]
        n37 = Index Array(array=w209, index=w213) -> (element=w211:i32)
        n38 = Add Array Elements(numeric array=w209) -> (sum=w208:i32)
        n39 = case shown="\"<\", Default" w212 {
          tunnel: w211 -> [w219 w222]
          tunnel: w210 -> [w218 w221]
          tunnel: [w217 w220] -> w205
          frame "<", Default {
            n40 = Greater?(x=w218, y=w219) -> (0:w217:bool)
          }
          frame ">" {
            n41 = Less?(x=w221, y=w222) -> (x < y?=w220:bool)
          }
        }
        n42 = Select(t=w206, s=w205, f=w204) -> (s? t:f=w203:string)
        n43 = Equal?(x="A" ("element"), y=w203) -> (x = y?=w202:bool)
      }
      n44 = xnode "Match Regular Expression"("input string"=w73, "regular expression"="[A,R]") -> ("whole match"=w74:string)  [unwired: 4 in, 4 out]
      n45 = Empty String/Path?(string/path=w74) -> (empty?=w72:bool)
    }
  }
  n46 = Add Array Elements(numeric array=w2) -> (sum=→"Task 1":i32)
